vi "Get Size of Data from TD - Waveform SGL - Returns Correct Size.vi"() -> ()   [LabVIEW 2017, in "Composition.Tests.lvlib"]
uses:
  Composition.Tests.lvlib
  <vilib>/addons/_JKI Toolkits/Caraya/classes/Assert/Assert Equal Value_Variant.vi
  Composition/Composition.lvlib
  <vilib>/addons/_JKI Toolkits/Caraya/classes/Assert/Assert.lvclass
  <vilib>/addons/_JKI Toolkits/Caraya/classes/Test/Test.lvclass
panel:
  out "error out":errorcluster
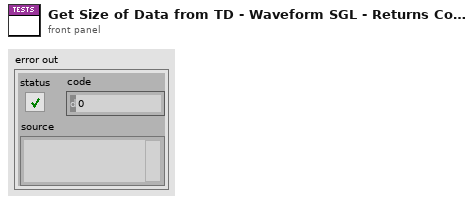
[diagram p1: front panel]
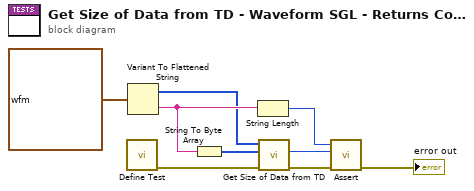
[diagram p0: block diagram]
diagram:
  n1 = call <vilib>:"Define Test.vi"() -> ("error out"=w5:errorcluster)  [unwired: 11 in]
  n2 = Variant To Flattened String(Variant=waveform(sgl) {"t0"=timestamp(0 s since 1904-01-01), "dt"=1.0, "Y"=[]}) -> (data string=w8:string, 1:w3:i16[])
  n3 = String To Byte Array(string=w8) -> (unsigned byte array=w1:u8[])
  n4 = String Length(string=w8) -> (length=w6:i32)
  n5 = call "Get Size of Data from TD.vi"("error in (no error)"=w5, "Data String"=w1, "Type Descriptor"=w3) -> ("error out"=w9:errorcluster, "Size of Data"=w2:i32)  [unwired: 7 in]
  n6 = call-poly <vilib>:"Assert.vi"("error in (no error)"=w9, "Y"=w2, "X"=w6) -> ("error out"=→"error out":errorcluster)  [unwired: 8 in]
